vi "CRYReport Function TX LIB.vi"(6 "Control Ref":refnum<k7>, 7 "sAction":string, 8 "nData":i32, 9 "sData":string, 10 "TXTextControl":refnum<k7>, 11 "cFrame":T1) -> (0 "nData_Out":i32, 1 "sData_Out":string, 3 "cFrame_Out":T1)   [LabVIEW 2013]
uses:
  CRYReport Global.vi
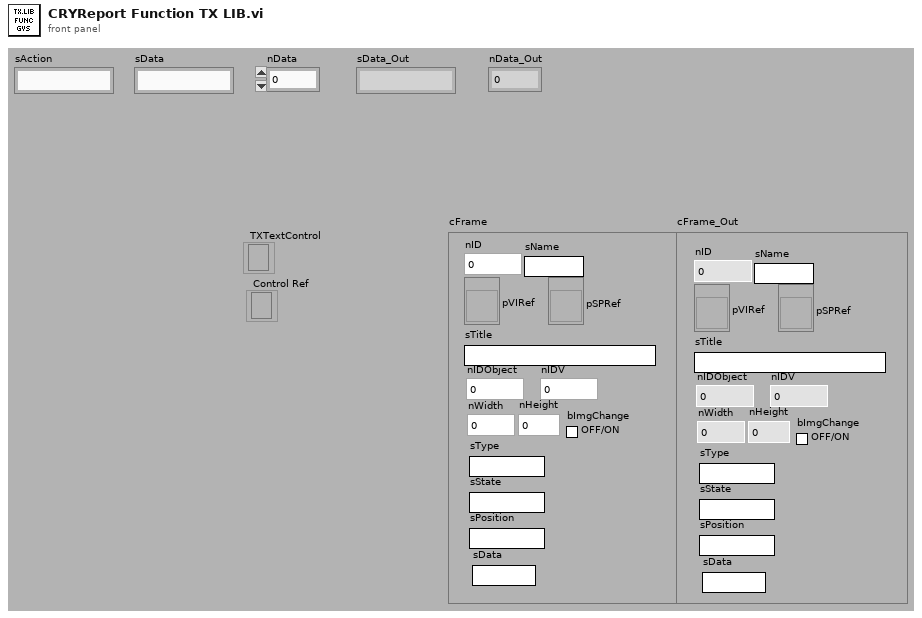
[diagram p1: front panel]
types:
  T1 = cluster{"nID":i16, "sName":string, "pVIRef":refnum<vi>, "pSPRef":refnum<vi>, "sTitle":string, "nIDObject":i16, "nIDV":i16, "nWidth":i16, "nHeight":i16, "bImgChange":bool, "sType":string, "sState":string, "sPosition":string, "sData":string}
  T2 = cluster{"nID":i32, "sName":string, "sType":string, "sProperty":string, "sTemplet":string, "sDocking":string, "pVIRef":refnum<vi>, "pSPRef":refnum<vi>, "pRefTemplet":refnum<vi>, "pRefSplitter":refnum<vi>[], "nPosSplitter":i32[], "pRefSP":refnum<vi>[], "nSPID":i32[], "sSPDock":string[], "nIDFrame":i32[], "nIDPanel":i32[], "nActiveFrame":i32, "nCountFrame":i32, "cFrame":cluster{"nID":i32, "sName":string, "sType":string, "sTitle":string, "sIcon":string, "pVIRef":refnum<vi>, "pSPRef":refnum<vi>, "cWiin":cluster{"sName":string, "sType":string, "pVIRef":refnum<vi>, "sData":string}, "cTab":cluster{"sTitle":string, "sIcon":string, "pSpliter":refnum<vi>, "nAvtivePage":i32, "nIDPage":i32[], "nIDFrame":i32[]}, "sData":string}[], "sData":string, "sSplitterName":string[]}
  T3 = cluster{"nCount":i16, "cFrameList":cluster{"nID":i16, "sName":string, "pVIRef":refnum<vi>, "pSPRef":refnum<vi>, "sTitle":string, "nIDObject":i16, "nIDV":i16, "nWidth":i16, "nHeight":i16, "bImgChange":bool, "sType":string, "sState":string, "sPosition":string, "sData":string}[], "sData":string}
  T4 = cluster{"nID":i16, "sName":string, "pVIRef":refnum<vi>, "pSPRef":refnum<vi>, "sTitle":string, "nIDObject":i16, "nIDV":i16, "nWidth":i16, "nHeight":i16, "bImgChange":bool, "sType":string, "sState":string, "sPosition":string, "sData":string}[]
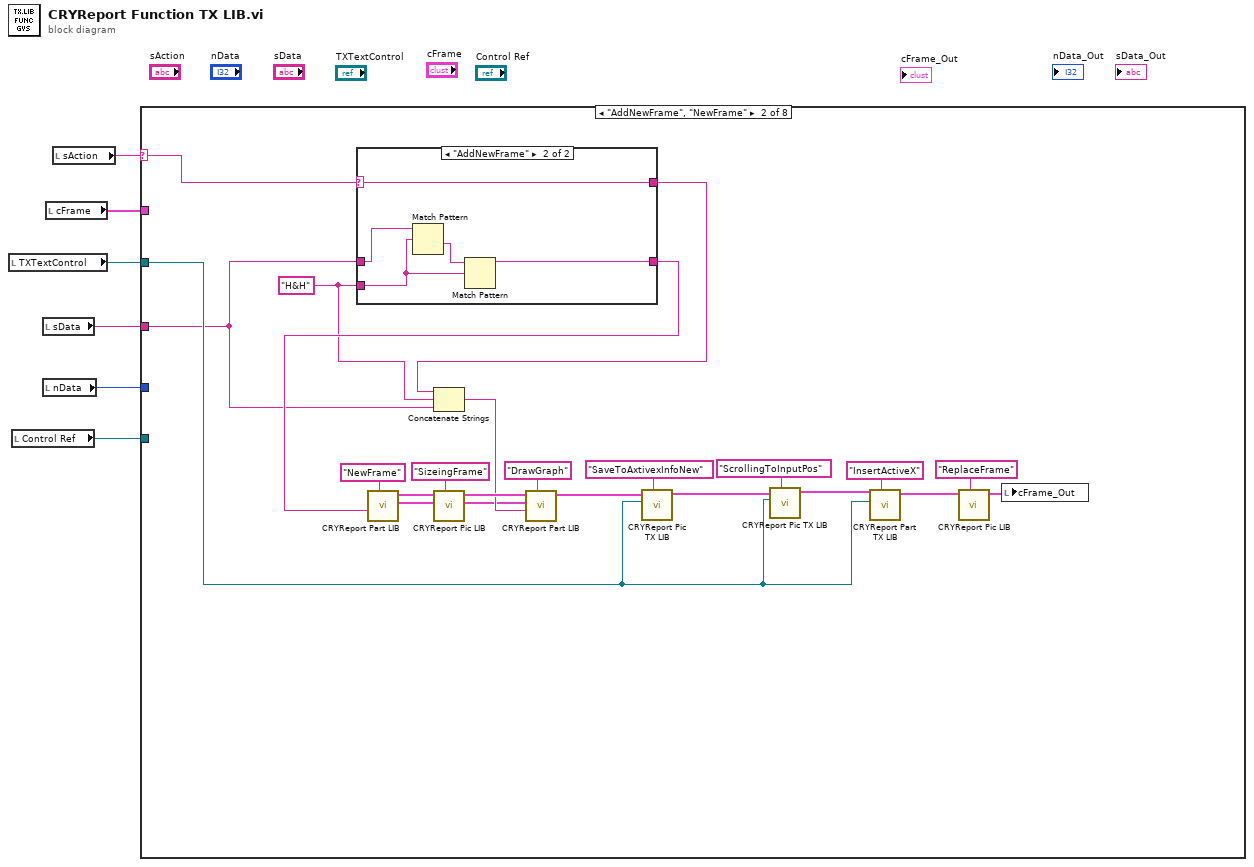
[diagram p0: block diagram]
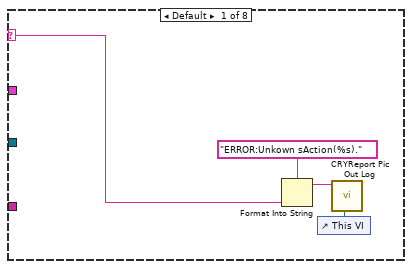
[diagram p2: hidden frame]
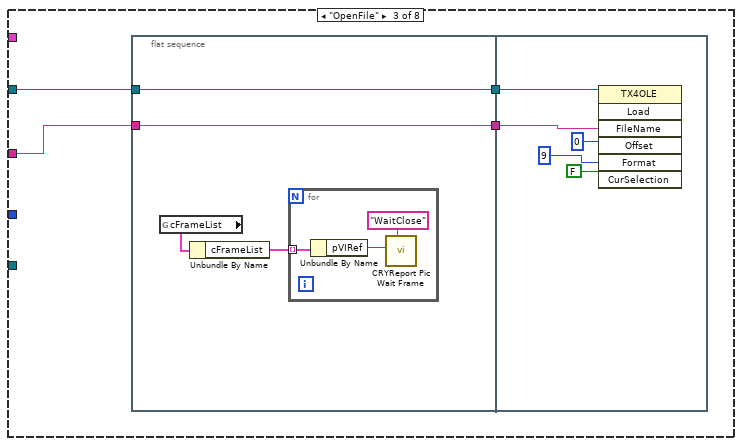
[diagram p4: hidden frame]
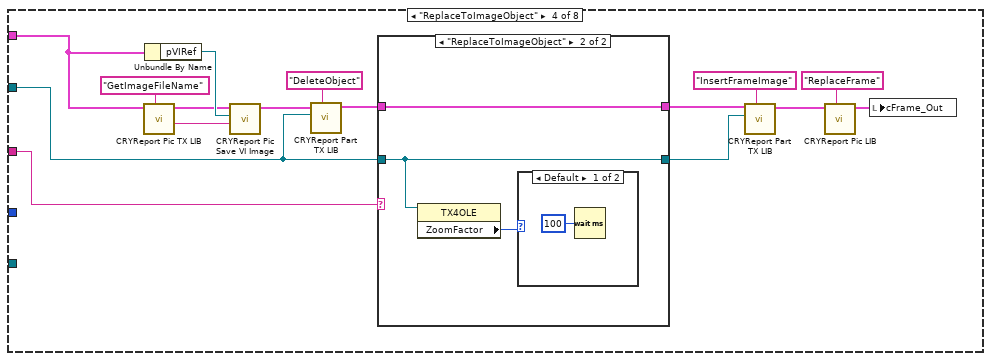
[diagram p5: hidden frame]
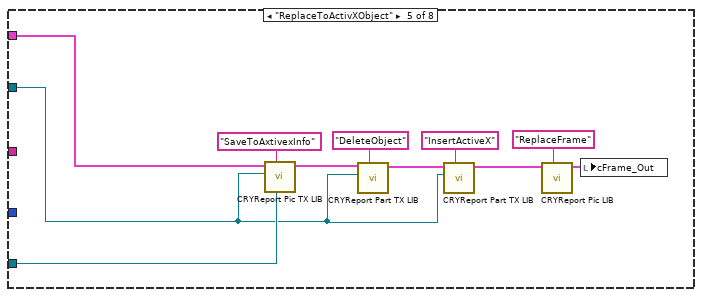
[diagram p8: hidden frame]
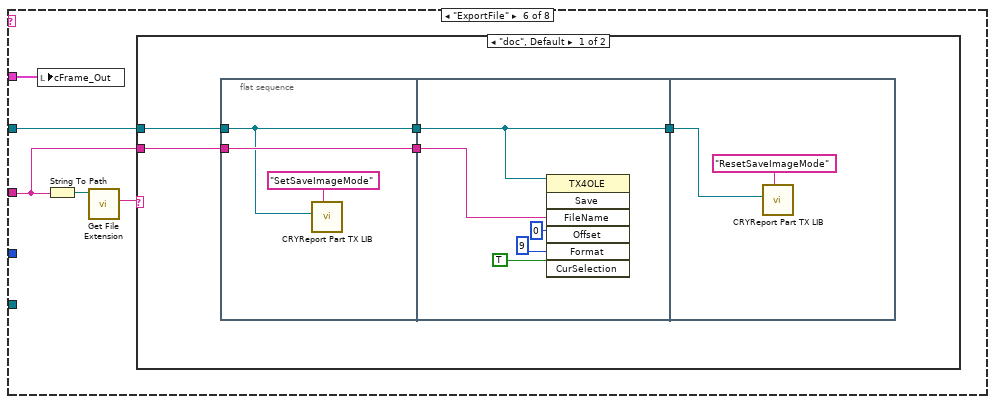
[diagram p9: hidden frame]
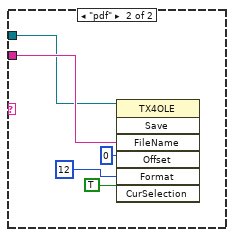
[diagram p10: hidden frame]
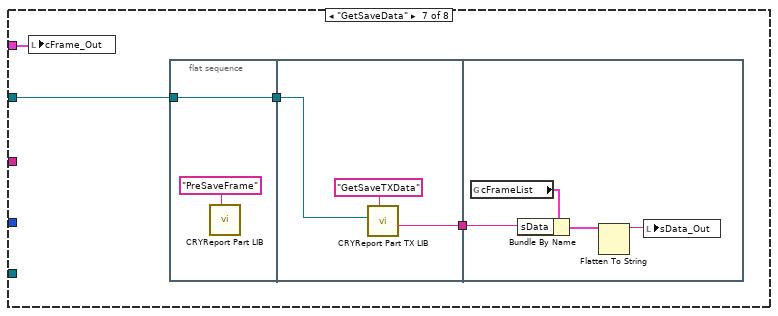
[diagram p11: hidden frame]
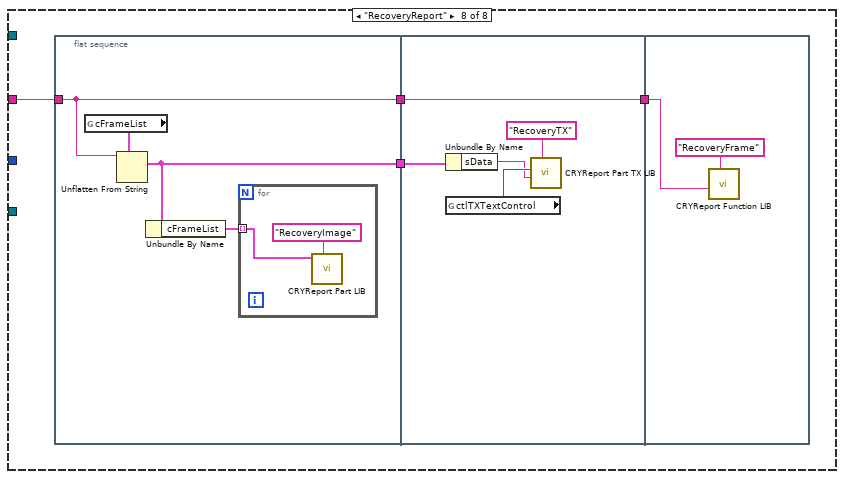
[diagram p12: hidden frame]
diagram:
  n1 = local read "TXTextControl"() -> (w2:refnum<k7>)
  n2 = local read "Control Ref"() -> (w1:refnum<k7>)
  n3 = local read "sData"() -> (w5:string)
  n4 = local read "nData"() -> (w4:i32)
  n5 = local read "cFrame"() -> (w3:T1)
  n6 = local read "sAction"() -> (w6:string)
  n7 = case shown="\"AddNewFrame\", \"NewFrame\"" w6 {
    selector: w6 -> [w8 w15 _ _ _ _ _ _]
    tunnel: w5 -> [_ w17 w44 w61 _ w90 _ w131]
    tunnel: w4 -> [_ _ _ _ _ _ _ _]
    tunnel: w3 -> [_ _ _ w63 w88 w94 w115 _]
    tunnel: w2 -> [_ w20 w43 w58 w79 w91 w116 _]
    tunnel: w1 -> [_ _ _ _ w89 _ _ _]
    frame Default {
      n8 = Format Into String(format string="ERROR:Unkown sAction(%s).", w8) -> (resulting string=w7:string)  [unwired: 2 in, 1 out]
      n9 = control-ref of="This VI"() -> (w10:refnum<vi>)
      n10 = call "CRYReport Pic Out Log.vi"("vi reference"=w10, "sData"=w7) -> ()  [unwired: 10 in]
    }
    frame "AddNewFrame", "NewFrame" {
      w13 = "H&H"
      n11 = case shown="\"AddNewFrame\"" w15 {
        selector: w15 -> [w34 w36]
        tunnel: w17 -> [w35 w39]
        tunnel: [w35 w38] -> w18
        tunnel: [w34 w36] -> w14
        tunnel: w13 -> [_ w37]
        frame "NewFrame", Default {
        }
        frame "AddNewFrame" {
          n12 = Match Pattern(string=w39, regular expression=w37) -> (after substring=w40:string)  [unwired: 1 in, 3 out]
          n13 = Match Pattern(string=w40, regular expression=w37) -> (before substring=w38:string)  [unwired: 1 in, 3 out]
        }
      }
      n14 = call "CRYReport Part LIB.vi"("sAction"="NewFrame", "sData"=w18) -> ("cView_Out"=w12:T2, "cFrame_Out"=w32:T1)  [unwired: 6 in, 2 out]
      n15 = Concatenate Strings(w14, w13, w17) -> (w16:string)
      n16 = call "CRYReport Pic LIB.vi"("sAction"="SizeingFrame", "cView"=w12, "cFrame"=w32) -> ("cView_Out"=w11:T2, "cFrame_Out"=w30:T1)  [unwired: 5 in, 2 out]
      n17 = call "CRYReport Part LIB.vi"("sAction"="DrawGraph", "sData"=w16, "cView"=w11, "cFrame"=w30) -> ("cFrame_Out"=w24:T1)  [unwired: 4 in, 3 out]
      n18 = call "CRYReport Pic TX LIB.vi"("sAction"="SaveToAxtivexInfoNew", "TXTextControl"=w20, "cFrame"=w24) -> ("cFrame_Out"=w22:T1)  [unwired: 6 in, 2 out]
      n19 = call "CRYReport Pic TX LIB.vi"("sAction"="ScrollingToInputPos", "TXTextControl"=w20, "cFrame"=w22) -> ("cFrame_Out"=w21:T1)  [unwired: 6 in, 2 out]
      n20 = call "CRYReport Part TX LIB.vi"("sAction"="InsertActiveX", "TXTextControl"=w20, "cFrame"=w21) -> ("cFrame_Out"=w27:T1)  [unwired: 6 in, 2 out]
      n21 = call "CRYReport Pic LIB.vi"("sAction"="ReplaceFrame", "cFrame"=w27) -> ("cFrame_Out"=w23:T1)  [unwired: 6 in, 3 out]
      n22 = local write "cFrame_Out"(w23) -> ()
    }
    frame "OpenFile" {
      n23 = flat-sequence {
        tunnel: w43 -> [w47]
        tunnel: w44 -> [w48]
        tunnel: [w48] -> w42
        tunnel: [w47] -> w41
        tunnel: w42 -> [w53]
        tunnel: w41 -> [w52]
        frame #0 {
          n24 = global read "CRYReport Global.vi" "cFrameList"() -> (w45:T3)
          n25 = Unbundle By Name(w45) -> ("cFrameList"=w46:T4)
          n26 = for {
            tunnel: w46 -> [w50] mode=indexing
            n27 = Unbundle By Name(w50) -> ("pVIRef"=w49:refnum<vi>)
            n28 = call "CRYReport Pic Wait Frame.vi"("sAction"="WaitClose", "vi reference"=w49) -> ()  [unwired: 9 in, 1 out]
          }
        }
        frame #1 {
          n29 = invoke class="TX4OLE" method="Load"(reference=w52, "FileName"=w53, "Offset"=0, "Format"=9 ("nData"), "CurSelection"=FALSE) -> ()  [unwired: 2 in, 7 out]
        }
      }
    }
    frame "ReplaceToImageObject" {
      n30 = call "CRYReport Pic TX LIB.vi"("sAction"="GetImageFileName", "cFrame"=w63) -> ("sData_Out"=w65:string, "cFrame_Out"=w64:T1)  [unwired: 7 in, 1 out]
      n31 = Unbundle By Name(w63) -> ("pVIRef"=w67:refnum<vi>)
      n32 = call "CRYReport Pic Save VI Image.vi"("sData"=w65, "pVIRef"=w67, "cFrame"=w64) -> ("cFrame_Out"=w62:T1)  [unwired: 7 in, 1 out]
      n33 = call "CRYReport Part TX LIB.vi"("sAction"="DeleteObject", "TXTextControl"=w58, "cFrame"=w62) -> ("cFrame_Out"=w60:T1)  [unwired: 6 in, 2 out]
      n34 = case shown="\"ReplaceToImageObject\"" w61 {
        tunnel: w60 -> [w74 w77]
        tunnel: [w74 w77] -> w59
        tunnel: w58 -> [w73 w76]
        tunnel: [w73 w76] -> w57
        frame Default {
        }
        frame "ReplaceToImageObject" {
          n35 = property class="TX4OLE"(reference=w76) -> ("ZoomFactor"=w75:i16)  [unwired: 1 in, 2 out]
          n36 = case shown="Default" w75 {
            frame Default {
              n37 = Wait (ms)(milliseconds to wait=u32 100) -> ()  [unwired: 1 out]
            }
            frame 100 {
            }
          }
        }
      }
      n38 = call "CRYReport Part TX LIB.vi"("sAction"="InsertFrameImage", "TXTextControl"=w57, "cFrame"=w59) -> ("cFrame_Out"=w69:T1)  [unwired: 6 in, 2 out]
      n39 = call "CRYReport Pic LIB.vi"("sAction"="ReplaceFrame", "cFrame"=w69) -> ("cFrame_Out"=w68:T1)  [unwired: 6 in, 3 out]
      n40 = local write "cFrame_Out"(w68) -> ()
    }
    frame "ReplaceToActivXObject" {
      n41 = call "CRYReport Pic TX LIB.vi"("Control Ref"=w89, "sAction"="SaveToAxtivexInfo", "TXTextControl"=w79, "cFrame"=w88) -> ("cFrame_Out"=w86:T1)  [unwired: 5 in, 2 out]
      n42 = call "CRYReport Part TX LIB.vi"("sAction"="DeleteObject", "TXTextControl"=w79, "cFrame"=w86) -> ("cFrame_Out"=w82:T1)  [unwired: 6 in, 2 out]
      n43 = call "CRYReport Part TX LIB.vi"("sAction"="InsertActiveX", "TXTextControl"=w79, "cFrame"=w82) -> ("cFrame_Out"=w81:T1)  [unwired: 6 in, 2 out]
      n44 = call "CRYReport Pic LIB.vi"("sAction"="ReplaceFrame", "cFrame"=w81) -> ("cFrame_Out"=w80:T1)  [unwired: 6 in, 3 out]
      n45 = local write "cFrame_Out"(w80) -> ()
    }
    frame "ExportFile" {
      n46 = local write "cFrame_Out"(w94) -> ()
      n47 = String To Path(string=w90) -> (path=w93:path)
      n48 = call <vilib>:"Get File Extension.vi"("file"=w93) -> ("lowercase file extension"=w92:string)  [unwired: 1 in, 9 out]
      n49 = case shown="\"doc\", Default" w92 {
        tunnel: w90 -> [w98 w111]
        tunnel: w91 -> [w99 w110]
        frame "doc", Default {
          n50 = flat-sequence {
            tunnel: w98 -> [w102]
            tunnel: w99 -> [w101]
            tunnel: [w101] -> w97
            tunnel: [w102] -> w96
            tunnel: w97 -> [w103]
            tunnel: w96 -> [w104]
            tunnel: [w103] -> w95
            tunnel: w95 -> [w108]
            frame #0 {
              n51 = call "CRYReport Part TX LIB.vi"("sAction"="SetSaveImageMode", "TXTextControl"=w101) -> ()  [unwired: 7 in, 3 out]
            }
            frame #1 {
              n52 = invoke class="TX4OLE" method="Save"(reference=w103, "FileName"=w104, "Offset"=0, "Format"=9, "CurSelection"=TRUE) -> ()  [unwired: 2 in, 7 out]
            }
            frame #2 {
              n53 = call "CRYReport Part TX LIB.vi"("sAction"="ResetSaveImageMode", "TXTextControl"=w108) -> ()  [unwired: 7 in, 3 out]
            }
          }
        }
        frame "pdf" {
          n54 = invoke class="TX4OLE" method="Save"(reference=w110, "FileName"=w111, "Offset"=0, "Format"=12, "CurSelection"=TRUE) -> ()  [unwired: 2 in, 7 out]
        }
      }
    }
    frame "GetSaveData" {
      n55 = local write "cFrame_Out"(w115) -> ()
      n56 = flat-sequence {
        tunnel: [w119] -> w117
        tunnel: w116 -> [w119]
        tunnel: [w122] -> w118
        tunnel: w117 -> [w121]
        tunnel: w118 -> [w126]
        frame #0 {
          n57 = call "CRYReport Part LIB.vi"("sAction"="PreSaveFrame") -> ()  [unwired: 7 in, 4 out]
        }
        frame #1 {
          n58 = call "CRYReport Part TX LIB.vi"("sAction"="GetSaveTXData", "TXTextControl"=w121) -> ("sData_Out"=w122:string)  [unwired: 7 in, 2 out]
        }
        frame #2 {
          n59 = global read "CRYReport Global.vi" "cFrameList"() -> (w127:T3)
          n60 = Bundle By Name(cluster=w127, "sData"=w126) -> (w125:T3)
          n61 = Flatten To String(anything=w125) -> (data string=w124:string)  [unwired: 3 in, 2 out]
          n62 = local write "sData_Out"(w124) -> ()
        }
      }
    }
    frame "RecoveryReport" {
      n63 = flat-sequence {
        tunnel: w131 -> [w134]
        tunnel: [w134] -> w129
        tunnel: [w133] -> w128
        tunnel: [w139] -> w130
        tunnel: w129 -> [w139]
        tunnel: w128 -> [w138]
        tunnel: w130 -> [w144]
        frame #0 {
          n64 = global read "CRYReport Global.vi" "cFrameList"() -> (w135:T3)
          n65 = Unflatten From String(type=w135, binary string=w134) -> (value=w133:T3)  [unwired: 3 in, 2 out]
          n66 = Unbundle By Name(w133) -> ("cFrameList"=w132:T4)
          n67 = for {
            tunnel: w132 -> [w136] mode=indexing
            n68 = call "CRYReport Part LIB.vi"("sAction"="RecoveryImage", "cFrame"=w136) -> ()  [unwired: 6 in, 4 out]
          }
        }
        frame #1 {
          n69 = Unbundle By Name(w138) -> ("sData"=w140:string)
          n70 = global read "CRYReport Global.vi" "ctlTXTextControl"() -> (w141:refnum<k7>)
          n71 = call "CRYReport Part TX LIB.vi"("sAction"="RecoveryTX", "sData"=w140, "TXTextControl"=w141) -> ()  [unwired: 6 in, 3 out]
        }
        frame #2 {
          n72 = call "CRYReport Function LIB.vi"("sAction"="RecoveryFrame", "sData"=w144) -> ()  [unwired: 6 in, 4 out]
        }
      }
    }
  }
